vi "add_subVI_node.vi"(8 "error in":errorcluster, 9 "ControlPaths":path, 10 "ControlPosition":cluster{"Left":i32, "Top":i32}, 11 "VI Ref In":refnum<vi>) -> (0 "error out":errorcluster, 2 "SubVI Refnum Out":refnum<vi>, 3 "VI Ref Out":refnum<vi>)   [LabVIEW 2018]
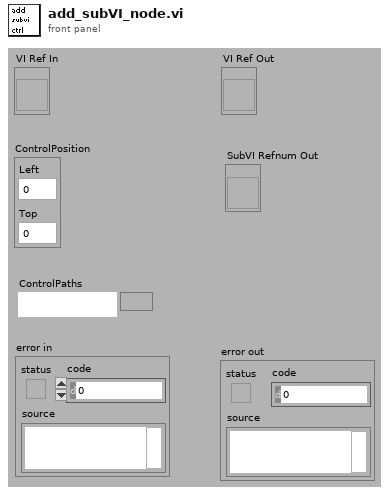
[diagram p1: front panel]
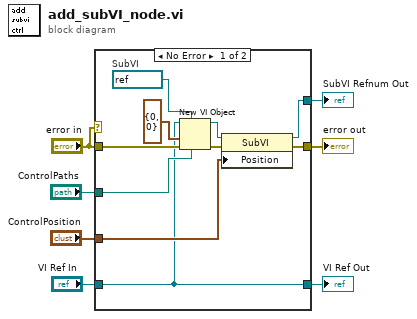
[diagram p0: block diagram]
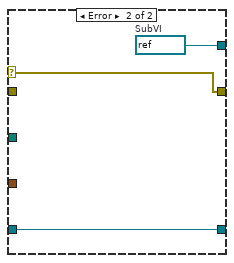
[diagram p2: hidden frame]
diagram:
  n1 = case shown="No Error" "error in" {
    selector: "error in" -> [_ w20]
    tunnel: "ControlPosition" -> [w17 _]
    tunnel: "VI Ref In" -> [w10 w19]
    tunnel: "ControlPaths" -> [w12 _]
    tunnel: "error in" -> [w11 _]
    tunnel: [w9 w20] -> w4
    tunnel: [w10 w19] -> w2
    tunnel: [w8 w18] -> w1
    frame No Error {
      w16 = refnum<vi> refnum  # SubVI
      n2 = New VI Object(vi object class=w16, owner refnum=w10, position/next to=cluster{"Horizontal":i16, "Vertical":i16} {"Horizontal"=0, "Vertical"=0}, 6:w12, 8:w11) -> (object refnum=w14:refnum<vi>, 0:w13:errorcluster)  [unwired: 1 in, 2 out]
      n3 = property class="SubVI"(reference=w14, error in=w13, "Position"=w17) -> (reference out=w8:refnum<vi>, error out=w9:errorcluster)
    }
    frame Error {
      w18 = refnum<vi> refnum  # SubVI
    }
  }
  "error out" <- w4
  "VI Ref Out" <- w2
  "SubVI Refnum Out" <- w1
